vi "FdxLogoutCvi.vi"(8 "error in":errorcluster, 11 "InstrumentHandle":u32) -> (0 "error out":errorcluster)   [LabVIEW 2020, in "AIM664LV.lvlib"]
doc: "This function closes the application interface for the specified resource and must be called last in an application program for all opened resources. After calling this function the handle is invalid and it is not possible to use it for further function calls."
uses:
  AIM664LV.lvlib
  FdxGlobalDllPath.vi
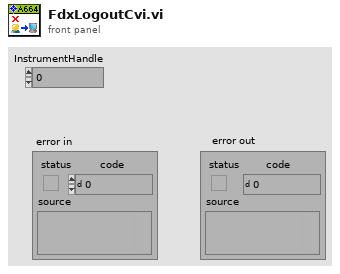
[diagram p1: front panel]
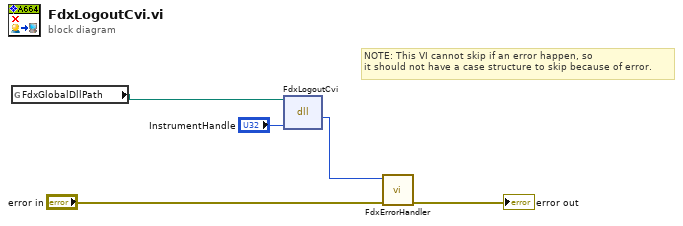
[diagram p0: block diagram]
diagram:
  # "NOTE: This VI cannot skip if an error happen, so\nit should not have a case structure to skip because of error."
  n1 = global read "FdxGlobalDllPath.vi" "FdxGlobalDllPath"() -> (w3:path)
  n2 = dll-call lib="aim_fdx.19.dll" fn="FdxLogoutCvi"(path in=w3, "Handle"="InstrumentHandle") -> ("status"=w2:i32)  [unwired: 3 in, 2 out]
  n3 = call "FdxErrorHandler.vi"("error in"="error in", "AIM Error"=w2) -> ("error out"=→"error out":errorcluster)  [unwired: 9 in]
